vi "New Progress Window.vi"(8 "error in (no error)":errorcluster) -> (0 "error out":errorcluster, 3 "progress queue":refnum<queue>)   [LabVIEW 2017, in "DSF System Explorer.lvlib"]
uses:
  DSF System Explorer.lvlib
  progress window data.ctl
  Progress Window.vi
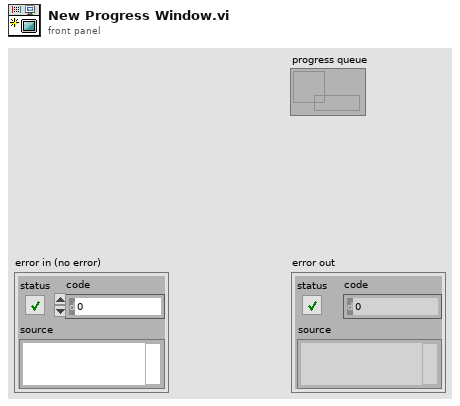
[diagram p1: front panel]
types:
  T1 = typedef "DSF System Explorer.lvlib/progress window data.ctl" = cluster{"stop":bool, "message":string, "progress":dbl}
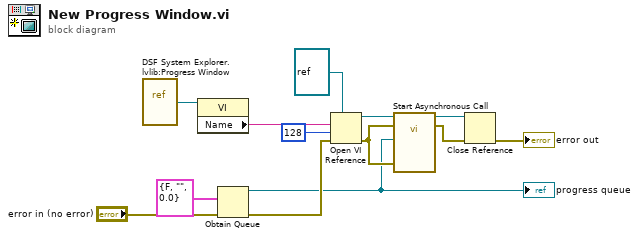
[diagram p0: block diagram]
diagram:
  n1 = vi-ref "DSF System Explorer.lvlib:Progress Window.vi"() -> (w12:refnum<vi>)
  n2 = property class="VI"(reference=w12) -> ("Name"=w11:string)  [unwired: 1 in, 2 out]
  n3 = Obtain Queue(element data type=T1 {"stop"=FALSE, "message"="", "progress"=0.0}, error in (no error)="error in (no error)") -> (queue out=w1:refnum<queue>, error out=w9:errorcluster)  [unwired: 3 in, 1 out]
  "progress queue" <- w1
  n4 = Open VI Reference(type specifier VI Refnum (for type only)=refnum<vi> refnum, vi path=w11, options=128, error in (no error)=w9) -> (vi reference=w7:refnum<vi>, error out=w6:errorcluster)  [unwired: 2 in]
  n5 = call-by-ref "Start Asynchronous Call"(reference=w7, error in=w6, 8:"error in (no error)"=w6, "queue"=w1) -> (reference out=w4:refnum<vi>, error out=w5:errorcluster)  [unwired: 9 in, 1 out]
  n6 = Close Reference(reference=w4, error in (no error)=w5) -> (error out=→"error out":errorcluster)
